vi "WaitTillWavelengthIsSetAndShowUserActions.vi"(11 "Topas":refnum<k24>) -> (3 "Topas Out":refnum<k24>)   [LabVIEW 2017]
uses:
  E:/UPWORK/Laser Tool/Laser/Topas/Topas4PublicAPI-master/NET_SDK/Topas4Lib.dll
  NET_SDK/Topas4Lib.dll
panel:
  in  "OK Button":bool
  out "Wavelength setting progress":dbl(slide) scale=0.0..1.0
  out "User Actions":string
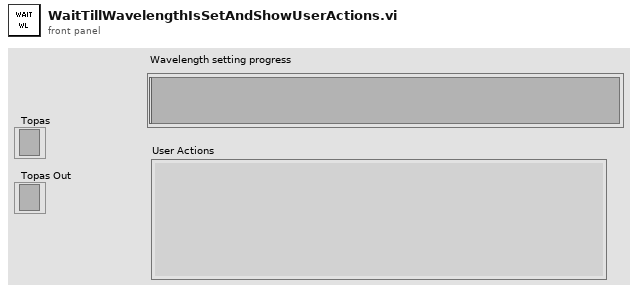
[diagram p1: front panel]
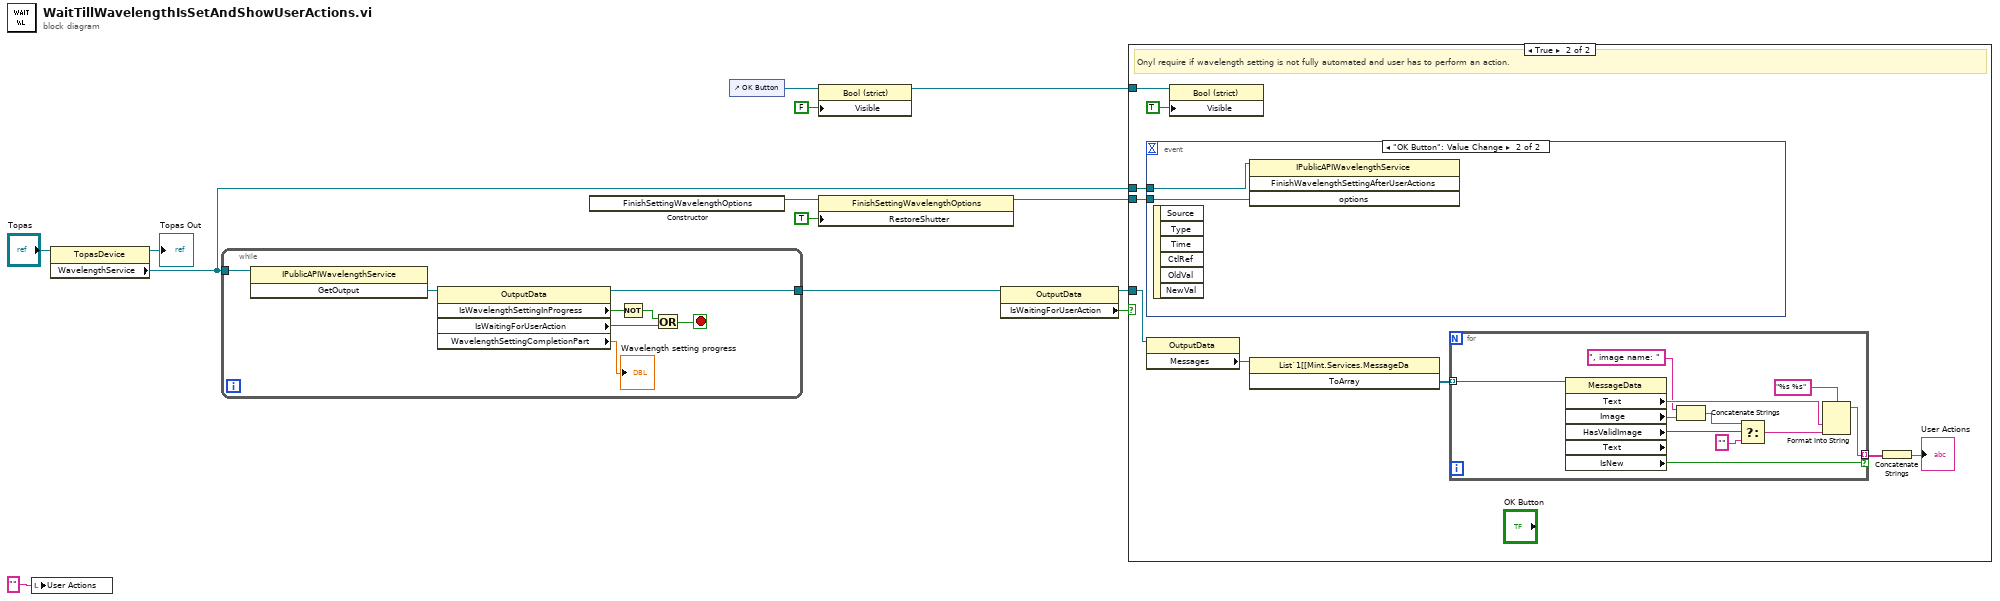
[diagram p0: block diagram]
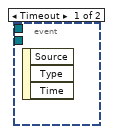
[diagram p3: hidden frame]
diagram:
  n1 = local write "User Actions"("" ("User Actions")) -> ()
  n2 = property class="TopasDevice"(reference="Topas") -> (reference out=→"Topas Out":refnum<k24>, "WavelengthService"=w9:refnum<k24>)  [unwired: 1 in, 1 out]
  n3 = while {
    tunnel: w9 -> [w21]
    tunnel: [w14] -> w12
    stop <- w16 stop-if-true
    n4 = invoke class="IPublicAPIWavelengthService" method="GetOutput"(reference=w21) -> ("GetOutput"=w20:refnum<k24>)  [unwired: 2 in, 2 out]
    n5 = property class="OutputData"(reference=w20) -> (reference out=w14:refnum<k24>, "IsWavelengthSettingInProgress"=w17:bool, "IsWaitingForUserAction"=w18:bool, "WavelengthSettingCompletionPart"=→"Wavelength setting progress":dbl)  [unwired: 1 in, 1 out]
    n6 = Not(x=w17) -> (.not. x?=w19:bool)
    n7 = Or(x=w19, y=w18) -> (x .or. y?=w16:bool)
  }
  n8 = constructor class="FinishSettingWavelengthOptions"() -> (reference out=w8:refnum<k24>)  [unwired: 3 in, 2 out]
  n9 = control-ref of="OK Button"() -> (w5:refnum<vi>)
  n10 = property class="Bool (strict)"(reference=w5, "Visible"=FALSE) -> (reference out=w3:refnum<vi>)  [unwired: 1 in, 1 out]
  n11 = property class="FinishSettingWavelengthOptions"(reference=w8, "RestoreShutter"=TRUE) -> (reference out=w6:refnum<k24>)  [unwired: 1 in, 1 out]
  n12 = property class="OutputData"(reference=w12) -> (reference out=w1:refnum<k24>, "IsWaitingForUserAction"=w13:bool)  [unwired: 1 in, 1 out]
  n13 = case shown="True" w13 {
    tunnel: w9 -> [_ w23]
    tunnel: w6 -> [_ w27]
    tunnel: w3 -> [_ w25]
    tunnel: w1 -> [_ w22]
    frame False {
    }
    frame True {
      # "Onyl require if wavelength setting is not fully automated and user has to perform an action."
      n14 = event shown="[1] \"OK Button\": Value Change" {
        selector: _ -> [_ _]
        dyn-events: _ -> [_ _]
        timeout: _ -> [_ _]
        tunnel: w23 -> [_ w32]
        tunnel: w27 -> [_ w31]
        event Timeout {
          n15 = event-data() -> ()  [unwired: 1 in, 3 out]
        }
        event "OK Button": Value Change {
          n16 = event-data() -> ()  [unwired: 1 in, 6 out]
          n17 = invoke class="IPublicAPIWavelengthService" method="FinishWavelengthSettingAfterUserActions"(reference=w32, "options"=w31) -> ()  [unwired: 2 in, 4 out]
        }
      }
      n18 = property class="OutputData"(reference=w22) -> ("Messages"=w24:refnum<k24>)  [unwired: 1 in, 2 out]
      n19 = property class="Bool (strict)"(reference=w25, "Visible"=TRUE) -> ()  [unwired: 1 in, 2 out]
      n20 = invoke class="List`1[[Mint.Services.MessageDa" method="ToArray"(reference=w24) -> ("ToArray"=w30:refnum<k24>[])  [unwired: 2 in, 2 out]
      n21 = for {
        tunnel: w30 -> [w43] mode=indexing
        tunnel: [w40] -> w29 mode=indexing if=w39
        n22 = property class="MessageData" props=["Text", "Image", "HasValidImage", "Text", "IsNew"](reference=w43) -> ("Text"=w36:string, "Image"=w34:string, "HasValidImage"=w42:bool, "IsNew"=w39:bool)  [unwired: 1 in, 3 out]
        n23 = Concatenate Strings(", image name: " ("string"), w34) -> (w33:string)
        n24 = Select(t=w33, s=w42, f="") -> (s? t:f=w37:string)
        n25 = Format Into String(format string="%s %s", w36, w37) -> (resulting string=w40:string)  [unwired: 2 in, 1 out]
      }
      n26 = Concatenate Strings(w29) -> (→"User Actions":string)
    }
  }
